vi "Get Ignore Tokens.vi"(8 "Error In":errorcluster, 11 "Ignore String":string) -> (0 "ErrorOut":errorcluster, 3 "Ignore Tokens":string[](array[string]))   [LabVIEW 2011, in "LVH-Build-Tools.lvlib"]
uses:
  LVH-Build-Tools.lvlib
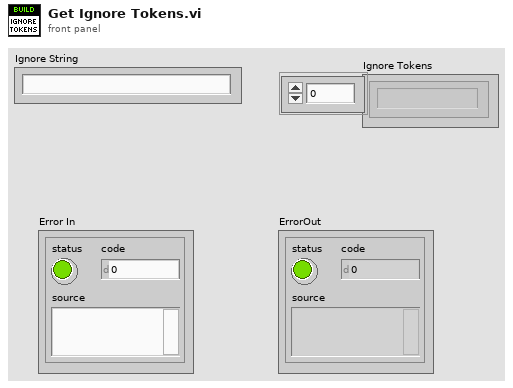
[diagram p1: front panel]
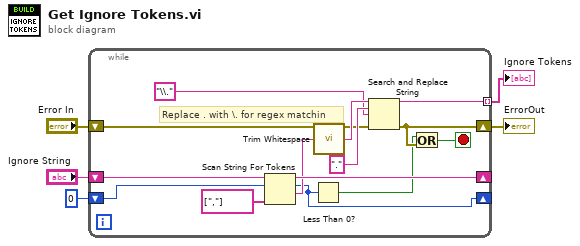
[diagram p0: block diagram]
diagram:
  n1 = while {
    shift-right: [w6] -> _
    shift-left: 0 ("offset") -> [w18]
    tunnel: [w10] -> w4 mode=indexing
    shift-right: [w15] -> _
    shift-left: "Ignore String" -> [w16]
    shift-right: [w8] -> w2
    shift-left: "Error In" -> [w9]
    stop <- w17 stop-if-true
    # "Replace . with \\. for regex matchin"
    n2 = Scan String For Tokens(6:string[] [","] ("delimiters (\\s,\\t,\\r,\\n)"), 8:w18, 9:w16) -> (1:w14:string, 2:w6:i32, 3:w15:string)  [unwired: 3 in, 1 out]
    n3 = Less Than 0?(x=w6) -> (x < 0?=w7:bool)
    n4 = call <vilib>:"Trim Whitespace.vi"("string"=w14) -> ("trimmed string"=w13:string)  [unwired: 1 in]
    n5 = Search and Replace String(input string=w13, search string=".", replace string="\\." ("replace string (\"\")"), error in=w9) -> (result string=w10:string, error out=w8:errorcluster)  [unwired: 4 in, 2 out]
    n6 = Or(x=w7, y=w8) -> (x .or. y?=w17:bool)
  }
  "Ignore Tokens" <- w4
  "ErrorOut" <- w2
